vi "Get System Image (File).vi"(4 "File and Directory Blacklist":string[](array[string]), 5 "Encryption Passphrase":string, 6 "Overwrite (F)":bool, 7 "Restart Automatically (T)":bool=TRUE, 8 "error in (no error)":errorcluster, 9 "Installed Software Only (F)":bool, 10 "Destination File":path, 11 "Session in":refnum<k21>) -> (0 "error out":errorcluster, 3 "Session out":refnum<k21>)   [LabVIEW 2012, in "nisyscfg.lvlib"]
doc: "Creates a system image file—a copy of the file contents on a primary hard drive of a system in zip format. The file is later applied to a system to restore it to the state captured on the image."
uses:
  <vilib>/nisyscfg/nisyscfg.lvlib
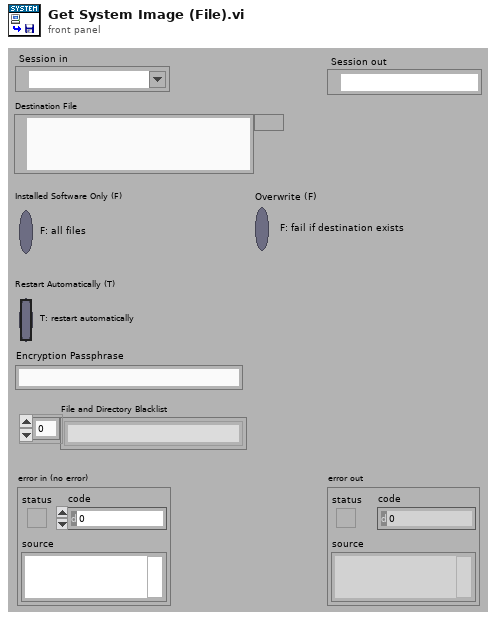
[diagram p1: front panel]
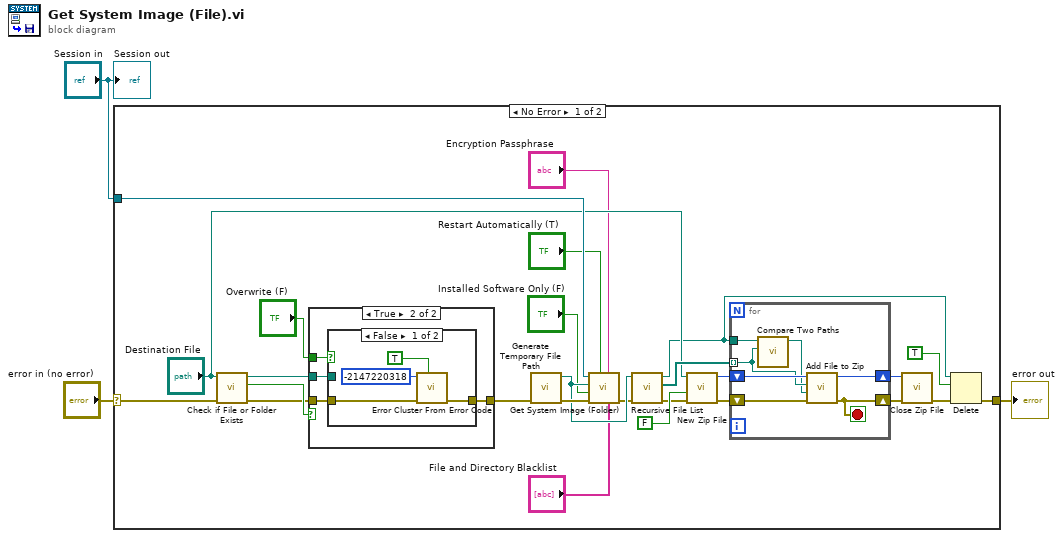
[diagram p0: block diagram]
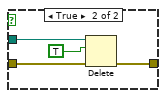
[diagram p3: hidden frame]
diagram:
  n1 = case shown="No Error" "error in (no error)" {
    selector: "error in (no error)" -> [w7 w50]
    tunnel: [w9 w50] -> w3
    tunnel: "Session in" -> [w23 _]
    frame No Error {
      n2 = call <vilib>:"Check if File or Folder Exists.vi"("error in (no error)"=w7, "path"="Destination File") -> ("error out"=w26:errorcluster, "file or folder exists?"=w29:bool, "dup path"=w27:path)  [unwired: 7 in]
      n3 = case shown="True" w29 {
        tunnel: "Overwrite (F)" -> [_ w41]
        tunnel: w27 -> [_ w40]
        tunnel: [w37 w39] -> w25
        tunnel: w26 -> [w37 w38]
        frame False {
        }
        frame True {
          n4 = case shown="False" w41 {
            tunnel: w40 -> [_ w49]
            tunnel: [w44 w47] -> w39
            tunnel: w38 -> [w45 w46]
            frame False {
              n5 = call <vilib>:"Error Cluster From Error Code.vi"("show call chain? (False)"=TRUE, "error in (no error)"=w45, "error code (0)"=-2147220318) -> ("error out"=w44:errorcluster)  [unwired: 6 in]
            }
            frame True {
              n6 = Delete(path (use dialog)=w49, entire hierarchy (F)=TRUE, error in=w46) -> (error out=w47:errorcluster)  [unwired: 2 in, 2 out]
            }
          }
        }
      }
      n7 = call <vilib>:"Generate Temporary File Path.vi"("error in (no error)"=w25) -> ("error out"=w24:errorcluster, "Unique Temporary File Path"=w14:path)  [unwired: 9 in]
      n8 = call <vilib>:"Get System Image (Folder).vi"("File and Directory Blacklist"="File and Directory Blacklist", "Encryption Passphrase"="Encryption Passphrase", "Restart Automatically (T)"="Restart Automatically (T)", "error in (no error)"=w24, "Installed Software Only (F)"="Installed Software Only (F)", "Destination Folder"=w14, "Session in"=w23) -> ("error out"=w13:errorcluster)  [unwired: 3 in, 1 out]
      n9 = call <vilib>:"Recursive File List.vi"("error in (no error)"=w13, "Folder Path"=w14) -> ("error out"=w18:errorcluster, "All Files in Dir"=w20:path[], "dup Folder Path"=w10:path)  [unwired: 1 in, 6 out]
      n10 = call <vilib>:"New Zip File.vi"("error in (no error)"=w18, "confirm overwrite? (F)"=FALSE, "target"="Destination File") -> ("error out"=w21:errorcluster, "zip file out"=w22:i64)  [unwired: 3 out]
      n11 = for {
        tunnel: w20 -> [w32] mode=indexing
        shift-right: [w34] -> w16
        shift-left: w22 -> [w36]
        shift-right: [w33] -> w17
        shift-left: w21 -> [w35]
        tunnel: w10 -> [w30]
        stop <- w33 stop-if-true
        n12 = call <vilib>:"Compare Two Paths.vi"("Path 2"=w32, "Path 1"=w30) -> ("Relative Path from 1 to 2"=w31:path)  [unwired: 1 in, 8 out]
        n13 = call <vilib>:"Add File to Zip.vi"("error in (no error)"=w35, "destination path in zip"=w31, "source file path"=w32, "zip file in"=w36) -> ("error out"=w33:errorcluster, "zip file out"=w34:i64)  [unwired: 6 out]
      }
      n14 = call <vilib>:"Close Zip File.vi"("error in (no error)"=w17, "zip file in"=w16) -> ("error out"=w12:errorcluster)  [unwired: 1 in, 4 out]
      n15 = Delete(path (use dialog)=w10, entire hierarchy (F)=TRUE, error in=w12) -> (error out=w9:errorcluster)  [unwired: 2 in, 2 out]
    }
    frame Error {
    }
  }
  "error out" <- w3
  "Session out" <- "Session in"
